vi "Widefield_globals.vi"() -> ()   [LabVIEW 2014]
panel:
  in  "Camera Type":u16(ring) items=["AVT Manta", "Hamamatsu Orca", "Photonfocus GigE", "Hamamatsu Orca2"]
  in  "FOV size":i32[](array[numeric])=[643, 394]
  in  "Binning":u16(ring) items=["1X1", "2X2", "4X4", "8X8"]
  in  "LED status":u16(ring) items=["All OFF", "IR LED", "Blue LED", "Green LED"]
  in  "conc mode":u16(ring) items=["normal"=0, "low"=1, "medium"=3, "high"=2, "highest"=4]
  in  "active cleaning":bool
  in  "Strobe order":bool
  in  "frame offset":u16
  in  "all stimuli":path[](array[path])=[path "C:/Documents and Settings/Florin/Desktop/testfolder/stimuli/4_0_1", path "C:/Documents and Settings/Florin/Desktop/testfolder/stimuli/4_0_2", path "C:/Documents and Settings/Florin/Desktop/testfolder/stimuli/4_1_3"]
  in  "camera resolution X,Y":i32[](array[numeric])=[640, 480]
  in  "projector resolution X,Y":i32[](array[numeric])=[643, 394]
  in  "roi_descript":path=path "C:/Documents and Settings/Florin/Desktop/testfolder/glom_descriptor"
  in  "Frame rate (Hz)":u16=25
  in  "LED settle":i32=500
  in  "Odor buildup":i32=125
  in  "Stimulus table":dbl[][](array[numeric])=[[1.0, 0.0, 0.0, 0.0, 0.0, 0.0, 0.0, 0.0], [3.0, 0.0, 0.0, 0.0, 0.0, 0.0, 0.0, 0.0], [5.0, 0.0, 0.0, 0.0, 0.0, 0.0, 0.0, 0.0], [7.0, 0.0, 0.0, 0.0, 0.0, 0.0, 0.0, 0.0], [9.0, 0.0, 0.0, 0.0, 0.0, 0.0, 0.0, 0.0]]
  in  "One Bulb?":bool
  in  "Pulsed?":bool
  in  "Projector":bool=TRUE
  out "Intrinsic":bool
  in  "Wavelength":u32=470
  in  "Igor Y Res":u32
  in  "Igor X Res":u32
  in  "IgorRes":bool
  out "Avg Image":u16[][](array[numeric])
  in  "WavelengthStr":string
  in  "AvgSubtract":bool
  in  "Palette":cluster{"R":u8, "G":u8, "B":u8}[](array[cluster])=[{"R"=0, "G"=0, "B"=0}, {"R"=0, "G"=0, "B"=0}, {"R"=0, "G"=0, "B"=0}, {"R"=0, "G"=0, "B"=0}, {"R"=0, "G"=0, "B"=0}, {"R"=0, "G"=0, "B"=0}, {"R"=0, "G"=0, "B"=0}, {"R"=0, "G"=0, "B"=0}, {"R"=0, "G"=0, "B"=0}, {"R"=0, "G"=0, "B"=0}, {"R"=0, "G"=0, "B"=0}, {"R"=0, "G"=0, "B"=0}, {"R"=0, "G"=0, "B"=0}, {"R"=0, "G"=0, "B"=0}, {"R"=0, "G"=0, "B"=0}, {"R"=0, "G"=0, "B"=0}, {"R"=0, "G"=0, "B"=80}, {"R"=0, "G"=0, "B"=80}, {"R"=0, "G"=0, "B"=80}, {"R"=0, "G"=0, "B"=80}, {"R"=0, "G"=0, "B"=80}, {"R"=0, "G"=0, "B"=80}, {"R"=0, "G"=0, "B"=80}, {"R"=0, "G"=0, "B"=80}, {"R"=0, "G"=0, "B"=80}, {"R"=0, "G"=0, "B"=80}, {"R"=0, "G"=0, "B"=80}, {"R"=0, "G"=0, "B"=80}, {"R"=0, "G"=0, "B"=80}, {"R"=0, "G"=0, "B"=80}, {"R"=0, "G"=0, "B"=80}, {"R"=0, "G"=0, "B"=80}, {"R"=0, "G"=0, "B"=160}, {"R"=0, "G"=0, "B"=160}, {"R"=0, "G"=0, "B"=160}, {"R"=0, "G"=0, "B"=160}, {"R"=0, "G"=0, "B"=160}, {"R"=0, "G"=0, "B"=160}, {"R"=0, "G"=0, "B"=160}, {"R"=0, "G"=0, "B"=160}, {"R"=0, "G"=0, "B"=160}, {"R"=0, "G"=0, "B"=160}, {"R"=0, "G"=0, "B"=160}, {"R"=0, "G"=0, "B"=160}, {"R"=0, "G"=0, "B"=160}, {"R"=0, "G"=0, "B"=160}, {"R"=0, "G"=0, "B"=160}, {"R"=0, "G"=0, "B"=160}, {"R"=0, "G"=0, "B"=254}, {"R"=0, "G"=0, "B"=254}, {"R"=0, "G"=0, "B"=254}, {"R"=0, "G"=0, "B"=254}, {"R"=0, "G"=0, "B"=254}, {"R"=0, "G"=0, "B"=254}, {"R"=0, "G"=0, "B"=254}, {"R"=0, "G"=0, "B"=254}, {"R"=0, "G"=0, "B"=254}, {"R"=0, "G"=0, "B"=254}, {"R"=0, "G"=0, "B"=254}, {"R"=0, "G"=0, "B"=254}, {"R"=0, "G"=0, "B"=254}, {"R"=0, "G"=0, "B"=254}, {"R"=0, "G"=0, "B"=254}, {"R"=0, "G"=0, "B"=254}, {"R"=0, "G"=80, "B"=0}, {"R"=0, "G"=80, "B"=0}, {"R"=0, "G"=80, "B"=0}, {"R"=0, "G"=80, "B"=0}, {"R"=0, "G"=80, "B"=0}, {"R"=0, "G"=80, "B"=0}, {"R"=0, "G"=80, "B"=0}, {"R"=0, "G"=80, "B"=0}, {"R"=0, "G"=80, "B"=0}, {"R"=0, "G"=80, "B"=0}, {"R"=0, "G"=80, "B"=0}, {"R"=0, "G"=80, "B"=0}, {"R"=0, "G"=80, "B"=0}, {"R"=0, "G"=80, "B"=0}, {"R"=0, "G"=80, "B"=0}, {"R"=0, "G"=80, "B"=0}, {"R"=0, "G"=160, "B"=0}, {"R"=0, "G"=160, "B"=0}, {"R"=0, "G"=160, "B"=0}, {"R"=0, "G"=160, "B"=0}, {"R"=0, "G"=160, "B"=0}, {"R"=0, "G"=160, "B"=0}, {"R"=0, "G"=160, "B"=0}, {"R"=0, "G"=160, "B"=0}, {"R"=0, "G"=160, "B"=0}, {"R"=0, "G"=160, "B"=0}, {"R"=0, "G"=160, "B"=0}, {"R"=0, "G"=160, "B"=0}, {"R"=0, "G"=160, "B"=0}, {"R"=0, "G"=160, "B"=0}, {"R"=0, "G"=160, "B"=0}, {"R"=0, "G"=160, "B"=0}, {"R"=0, "G"=254, "B"=0}, {"R"=0, "G"=254, "B"=0}, {"R"=0, "G"=254, "B"=0}, {"R"=0, "G"=254, "B"=0}, {"R"=0, "G"=254, "B"=0}, {"R"=0, "G"=254, "B"=0}, {"R"=0, "G"=254, "B"=0}, {"R"=0, "G"=254, "B"=0}, {"R"=0, "G"=254, "B"=0}, {"R"=0, "G"=254, "B"=0}, {"R"=0, "G"=254, "B"=0}, {"R"=0, "G"=254, "B"=0}, {"R"=0, "G"=254, "B"=0}, {"R"=0, "G"=254, "B"=0}, {"R"=0, "G"=254, "B"=0}, {"R"=0, "G"=254, "B"=0}, {"R"=0, "G"=160, "B"=80}, {"R"=0, "G"=160, "B"=80}, {"R"=0, "G"=160, "B"=80}, {"R"=0, "G"=160, "B"=80}, {"R"=0, "G"=160, "B"=80}, {"R"=0, "G"=160, "B"=80}, {"R"=0, "G"=160, "B"=80}, {"R"=0, "G"=160, "B"=80}, {"R"=0, "G"=160, "B"=80}, {"R"=0, "G"=160, "B"=80}, {"R"=0, "G"=160, "B"=80}, {"R"=0, "G"=160, "B"=80}, {"R"=0, "G"=160, "B"=80}, {"R"=0, "G"=160, "B"=80}, {"R"=0, "G"=160, "B"=80}, {"R"=0, "G"=160, "B"=80}, {"R"=0, "G"=160, "B"=160}, {"R"=0, "G"=160, "B"=160}, {"R"=0, "G"=160, "B"=160}, {"R"=0, "G"=160, "B"=160}, {"R"=0, "G"=160, "B"=160}, {"R"=0, "G"=160, "B"=160}, {"R"=0, "G"=160, "B"=160}, {"R"=0, "G"=160, "B"=160}, {"R"=0, "G"=160, "B"=160}, {"R"=0, "G"=160, "B"=160}, {"R"=0, "G"=160, "B"=160}, {"R"=0, "G"=160, "B"=160}, {"R"=0, "G"=160, "B"=160}, {"R"=0, "G"=160, "B"=160}, {"R"=0, "G"=160, "B"=160}, {"R"=0, "G"=160, "B"=160}, {"R"=0, "G"=160, "B"=254}, {"R"=0, "G"=160, "B"=254}, {"R"=0, "G"=160, "B"=254}, {"R"=0, "G"=160, "B"=254}, {"R"=0, "G"=160, "B"=254}, {"R"=0, "G"=160, "B"=254}, {"R"=0, "G"=160, "B"=254}, {"R"=0, "G"=160, "B"=254}, {"R"=0, "G"=160, "B"=254}, {"R"=0, "G"=160, "B"=254}, {"R"=0, "G"=160, "B"=254}, {"R"=0, "G"=160, "B"=254}, {"R"=0, "G"=160, "B"=254}, {"R"=0, "G"=160, "B"=254}, {"R"=0, "G"=160, "B"=254}, {"R"=0, "G"=160, "B"=254}, {"R"=0, "G"=254, "B"=160}, {"R"=0, "G"=254, "B"=160}, {"R"=0, "G"=254, "B"=160}, {"R"=0, "G"=254, "B"=160}, {"R"=0, "G"=254, "B"=160}, {"R"=0, "G"=254, "B"=160}, {"R"=0, "G"=254, "B"=160}, {"R"=0, "G"=254, "B"=160}, {"R"=0, "G"=254, "B"=160}, {"R"=0, "G"=254, "B"=160}, {"R"=0, "G"=254, "B"=160}, {"R"=0, "G"=254, "B"=160}, {"R"=0, "G"=254, "B"=160}, {"R"=0, "G"=254, "B"=160}, {"R"=0, "G"=254, "B"=160}, {"R"=0, "G"=254, "B"=160}, {"R"=0, "G"=254, "B"=254}, {"R"=0, "G"=254, "B"=254}, {"R"=0, "G"=254, "B"=254}, {"R"=0, "G"=254, "B"=254}, {"R"=0, "G"=254, "B"=254}, {"R"=0, "G"=254, "B"=254}, {"R"=0, "G"=254, "B"=254}, {"R"=0, "G"=254, "B"=254}, {"R"=0, "G"=254, "B"=254}, {"R"=0, "G"=254, "B"=254}, {"R"=0, "G"=254, "B"=254}, {"R"=0, "G"=254, "B"=254}, {"R"=0, "G"=254, "B"=254}, {"R"=0, "G"=254, "B"=254}, {"R"=0, "G"=254, "B"=254}, {"R"=0, "G"=254, "B"=254}, {"R"=160, "G"=254, "B"=0}, {"R"=160, "G"=254, "B"=0}, {"R"=160, "G"=254, "B"=0}, {"R"=160, "G"=254, "B"=0}, {"R"=160, "G"=254, "B"=0}, {"R"=160, "G"=254, "B"=0}, {"R"=160, "G"=254, "B"=0}, {"R"=160, "G"=254, "B"=0}, {"R"=160, "G"=254, "B"=0}, {"R"=160, "G"=254, "B"=0}, {"R"=160, "G"=254, "B"=0}, {"R"=160, "G"=254, "B"=0}, {"R"=160, "G"=254, "B"=0}, {"R"=160, "G"=254, "B"=0}, {"R"=160, "G"=254, "B"=0}, {"R"=160, "G"=254, "B"=0}, {"R"=160, "G"=254, "B"=254}, {"R"=160, "G"=254, "B"=254}, {"R"=160, "G"=254, "B"=254}, {"R"=160, "G"=254, "B"=254}, {"R"=160, "G"=254, "B"=254}, {"R"=160, "G"=254, "B"=254}, {"R"=160, "G"=254, "B"=254}, {"R"=160, "G"=254, "B"=254}, {"R"=160, "G"=254, "B"=254}, {"R"=160, "G"=254, "B"=254}, {"R"=160, "G"=254, "B"=254}, {"R"=160, "G"=254, "B"=254}, {"R"=160, "G"=254, "B"=254}, {"R"=160, "G"=254, "B"=254}, {"R"=160, "G"=254, "B"=254}, {"R"=160, "G"=254, "B"=254}, {"R"=254, "G"=0, "B"=0}, {"R"=254, "G"=0, "B"=0}, {"R"=254, "G"=0, "B"=0}, {"R"=254, "G"=0, "B"=0}, {"R"=254, "G"=0, "B"=0}, {"R"=254, "G"=0, "B"=0}, {"R"=254, "G"=0, "B"=0}, {"R"=254, "G"=0, "B"=0}, {"R"=254, "G"=0, "B"=0}, {"R"=254, "G"=0, "B"=0}, {"R"=254, "G"=0, "B"=0}, {"R"=254, "G"=0, "B"=0}, {"R"=254, "G"=0, "B"=0}, {"R"=254, "G"=0, "B"=0}, {"R"=254, "G"=0, "B"=0}, {"R"=254, "G"=0, "B"=0}, {"R"=254, "G"=0, "B"=80}, {"R"=254, "G"=0, "B"=160}, {"R"=254, "G"=0, "B"=254}, {"R"=254, "G"=0, "B"=254}, {"R"=254, "G"=80, "B"=254}, {"R"=254, "G"=80, "B"=254}, {"R"=254, "G"=80, "B"=254}, {"R"=254, "G"=80, "B"=254}, {"R"=254, "G"=80, "B"=254}, {"R"=254, "G"=160, "B"=254}, {"R"=254, "G"=166, "B"=254}, {"R"=254, "G"=176, "B"=254}, {"R"=254, "G"=186, "B"=254}, {"R"=254, "G"=196, "B"=254}, {"R"=254, "G"=236, "B"=254}, {"R"=254, "G"=254, "B"=254}]
  in  "ExposureTime":dbl=20.0
  in  "NumFramesDiscard":i32
  in  "Control LED?":bool
  in  "InterTrial Interval":i32=30000
  in  "Randomize?":bool
  in  "SingleFrames":bool=TRUE
  in  "Y Res":u32=256
  in  "X Res":u32=320
  in  "Y Binning":u32=4
  in  "X Binning":u32=4
  in  "TimeForFrame":u32=40
  in  "Camera":i32
  in  "File Path":path
  in  "Number of Odors":u32=5
  in  "# Repeats":u16=5
  # "Widefield Globals"
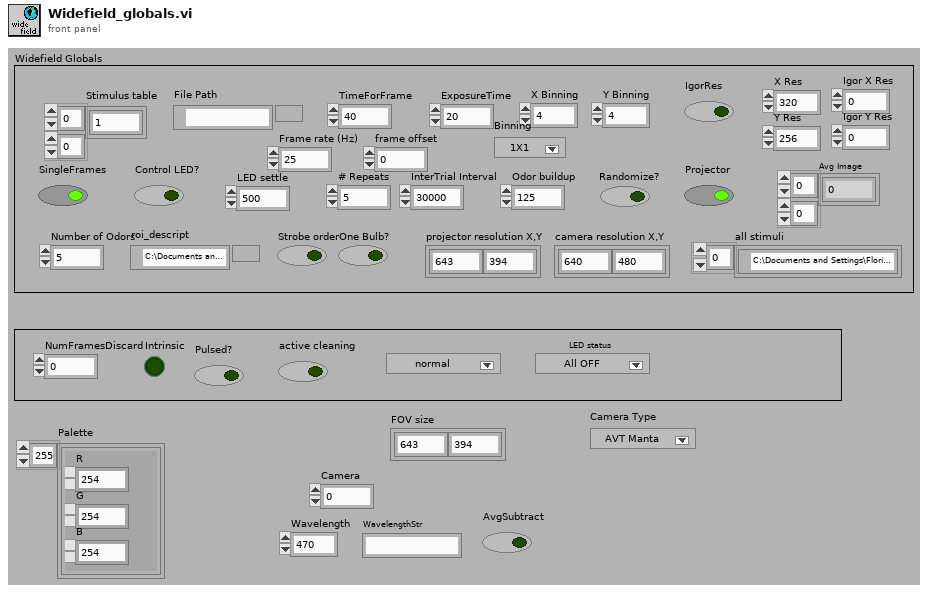
[diagram p1: front panel]
diagram:
